vi "GUI_StagingJetStages.vi"() -> ()   [LabVIEW 2013]
uses:
  shared programs/GUI_Template/GUI_master/tcp_new_data_event.ctl
  shared programs/GUI_Template/GUI_master/tcp new data cluster.ctl
panel:
  in  "stepsize::1":dbl=0.02 caption="stepsize" min=0.001 max=1.0
  in  "relativeMove.Axis 2neg::1":bool caption="-Y"
  in  "relativeMove.Axis 1neg::1":bool caption="-X"
  in  "relativeMove.Axis 2pos::1":bool caption="+Y"
  in  "relativeMove.Axis 1pos::1":bool caption="+X"
  in  "relativeMove.Axis 3neg::1":bool caption="-Z"
  in  "relativeMove.Axis 3pos::1":bool caption="+Z"
  in  "Status.Axis 3::1":u16(ring)=3 caption="Status" items=["Not referenced", "Homing", "Moving", "Ready"]
  in  "Position.Axis 3::1":dbl caption="Z" min=-12.0 max=12.0 format="%_4f"
  out "error IO 2":errorcluster
  out "tcp data event":T1
  out "GUIdevice 1":string="10TW_ESP"
  in  "Status.Axis 2::1":u16(ring)=3 caption="Status" items=["Not referenced", "Homing", "Moving", "Ready"]
  in  "Status.Axis 1::1":u16(ring)=3 caption="Staging Jet Stages" items=["Not referenced", "Homing", "Moving", "Ready"]
  in  "Position.Axis 2::1":dbl caption="Y" min=-12.0 max=12.0 format="%_4f"
  in  "stop":bool
  in  "Position.Axis 1::1":dbl caption="X" min=-12.0 max=12.0 format="%_4f"
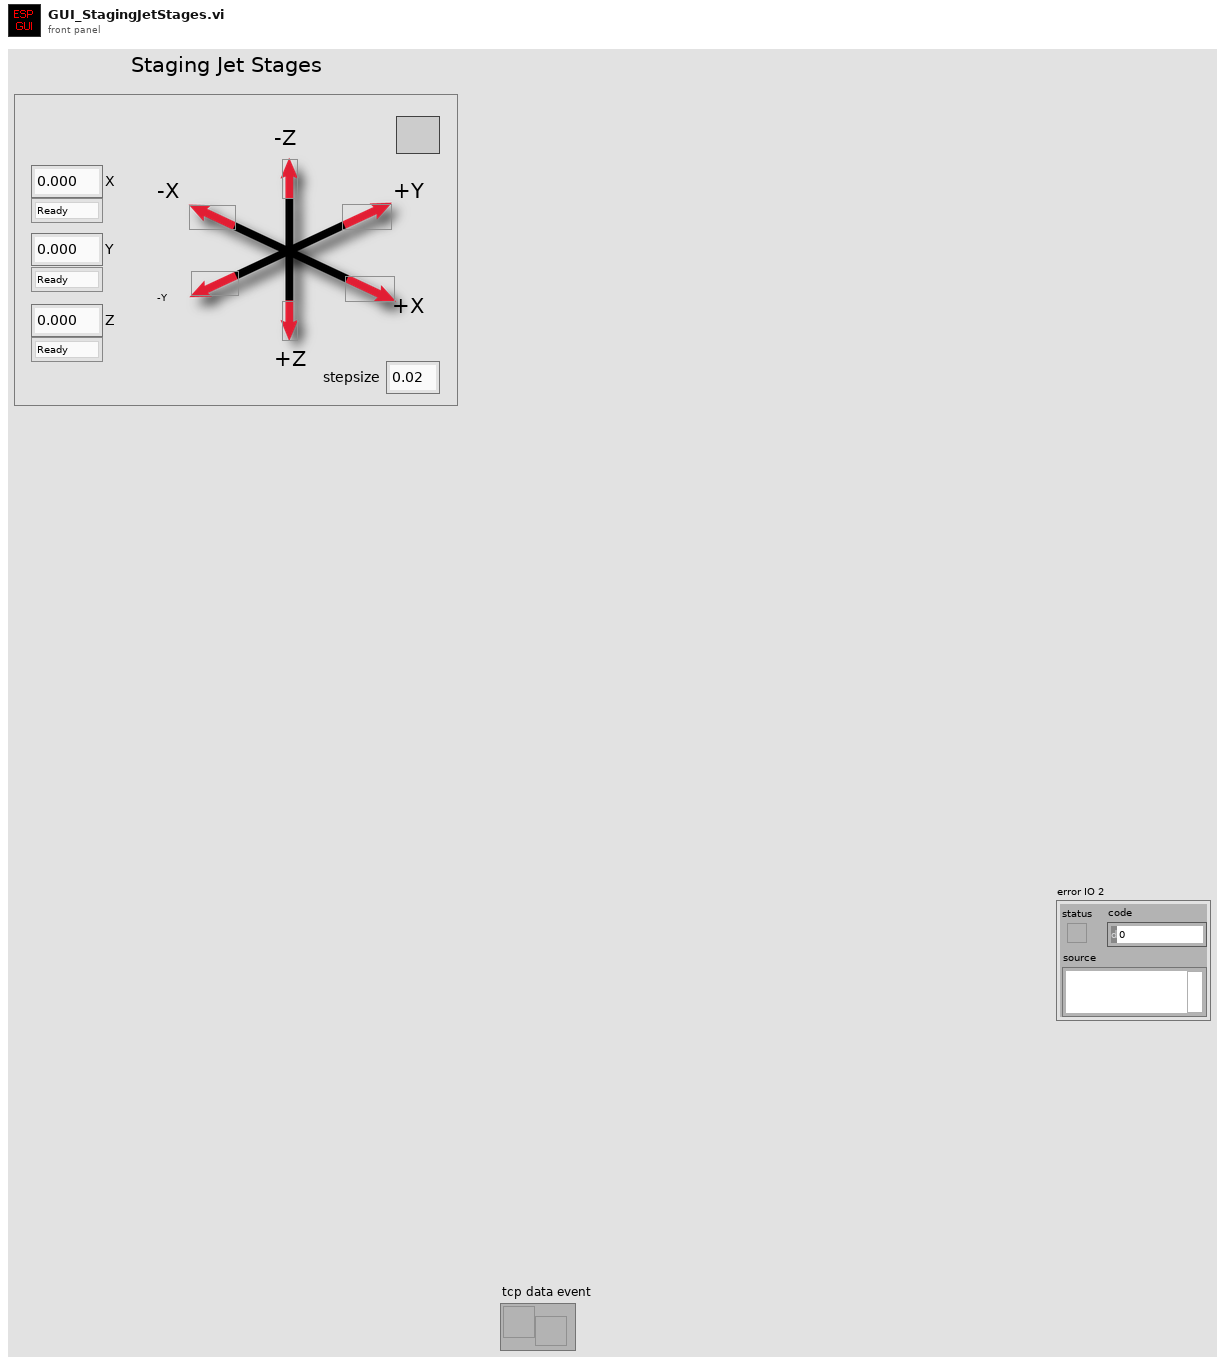
[diagram p1: front panel]
types:
  T1 = typedef "tcp_new_data_event.ctl" = refnum<user-event>
  T2 = typedef "tcp new data cluster.ctl" = cluster{"EventEnum":enum16{"new data", "connection status update"}, "Device name":string}
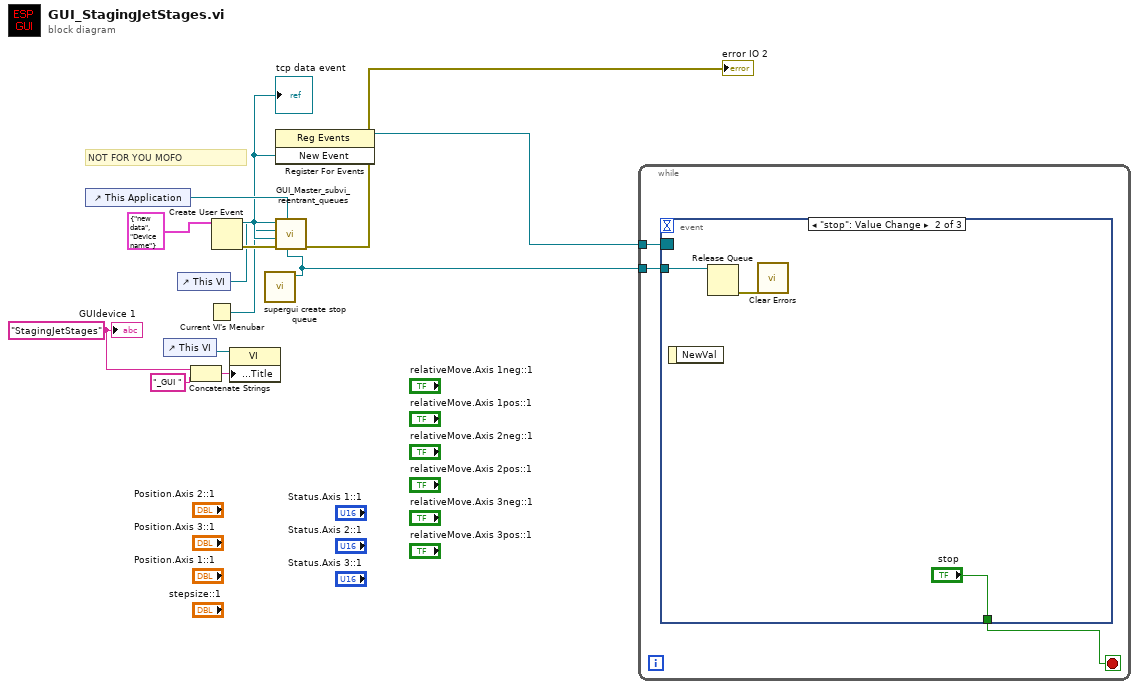
[diagram p0: block diagram]
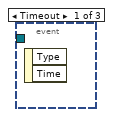
[diagram p2: hidden frame]
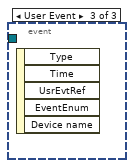
[diagram p3: hidden frame]
diagram:
  w1 = "StagingJetStages" ("GUIdevice 1")
  # "NOT FOR YOU MOFO"
  n1 = control-ref of="This Application"() -> (w13:refnum<vi>)
  n2 = control-ref of="This VI"() -> (w4:refnum<vi>)
  n3 = control-ref of="This VI"() -> (w8:refnum<vi>)
  n4 = Concatenate Strings(w1, "_GUI ") -> (w3:string)
  n5 = Current VI's Menubar() -> (w9:refnum<k9>)
  n6 = Create User Event(user event datatype=T2 {"EventEnum"=enum."new data", "Device name"="Device name"} ("New Event")) -> (user event=w12:refnum<user-event>, error out=w11:errorcluster)  [unwired: 1 in]
  "tcp data event" <- w12
  n7 = property class="VI"(reference=w4, "Front Panel.Title"=w3) -> ()  [unwired: 1 in, 2 out]
  n8 = call "supergui create stop queue.vi"() -> ("STOP Queue out"=w5:refnum<queue>)  [unwired: 11 in]
  n9 = register-events(w12) -> (reference out=w6:refnum<event-registration>)  [unwired: 2 in, 1 out]
  n10 = call "GUI_Master_subvi_reentrant_queues.vi"("STOP Queue in"=w5, "This Application"=w13, "error in (no error)"=w11, "tcp data event"=w12, "Caller menu reference"=w9, "Caller VI ref"=w8) -> ("error out"=→"error IO 2":errorcluster)  [unwired: 5 in]
  n11 = while {
    tunnel: w6 -> [w16]
    tunnel: w5 -> [w14]
    stop <- w15 stop-if-true
    n12 = event shown="[1] \"stop\": Value Change" {
      selector: w16 -> [_ _ _]
      dyn-events: _ -> [_ _ _]
      timeout: _ -> [_ _ _]
      tunnel: [_ "stop" _] -> w15
      tunnel: w14 -> [_ w18 _]
      event Timeout {
        n13 = event-data() -> ()  [unwired: 1 in, 2 out]
      }
      event "stop": Value Change {
        n14 = event-data() -> ()  [unwired: 1 in, 1 out]
        n15 = Release Queue(queue=w18) -> (error out=w17:errorcluster)  [unwired: 2 in, 2 out]
        n16 = call <vilib>:"Clear Errors.vi"("error in (no error)"=w17) -> ()  [unwired: 6 in, 1 out]
      }
      event User Event {
        n17 = event-data() -> ()  [unwired: 1 in, 5 out]
      }
    }
  }
  "GUIdevice 1" <- w1
